vi "Dashboard Main.vi"() -> ()   [LabVIEW 2019]
uses:
  <vilib>/Utility/miscctls.llb/LVRowAndColumnTypeDef.ctl
  <vilib>/event_ctls.llb/eventvkey.ctl
  <vilib>/Rock Robotics/Network Tables/NT Read Numeric Array.vi
  <vilib>/Rock Robotics/Network Tables/NT Read Boolean.vi
  <vilib>/Rock Robotics/WPI/Dashboard/WPI_DashboardLogging Global.vi
panel:
  in  "Camera Settings Right":T1={"Frame Rate"=30, "Compression"=30, "Size"=1, "DB Camera Config"=FALSE} {"Frame Rate" scale=1.0..30.0; "Compression" scale=100.0..-1.0; "Size" items=["640x480", "320x240", "160x120"]}
  in  "Camera Name Right":string(combo)="No Camera Selection"
  out "Camera Perf":string
  in  "Camera Settings":T1={"Frame Rate"=30, "Compression"=30, "Size"=1, "DB Camera Config"=FALSE} {"Frame Rate" scale=1.0..30.0; "Compression" scale=100.0..-1.0; "Size" items=["640x480", "320x240", "160x120"]}
  in  "TCP":refnum<k5>
  in  "Rec Mode":enum32{"Stop", "Record", "Playback"}(radio)
  out "Robot IP":string
  out "Image Message":string="Timeout in Camera Communications"
  in  "Dashboard Tab":T2(tab)=enum."Custom"
  in  "Select Auto":string(combo)="Select Autonomous ..."
  out "NT Connection":bool
  out "MotorChart R":cluster{"Numeric":dbl, "Numeric":dbl}(graph)
  out "MotorChart L":cluster{"Numeric":dbl, "Numeric":dbl}(graph)
  out "MotorSliders R":cluster{"MotorSlide1":dbl, "MotorSlide2":dbl} {"MotorSlide2" scale=-1.0..1.0 scale format="%#_2e"; "MotorSlide1" scale=-1.0..1.0 scale format="%#_2e"}
  out "MotorSliders L":cluster{"MotorSlide1":dbl, "MotorSlide2":dbl} {"MotorSlide2" scale=-1.0..1.0 scale format="%#_2e"; "MotorSlide1" scale=-1.0..1.0 scale format="%#_2e"}
  out "Gyro":dbl(knob) scale=0.0..360.0
  out "JS1 Z":dbl(slide) scale=-1.0..1.0 scale format="%#_2e"
  out "JS1 Graph":cluster{"X":dbl, "Y":dbl}[](graph)
  out "JS1 Buttons":T3
  out "JS2 Z":dbl(slide) scale=-1.0..1.0 scale format="%#_2e"
  out "JS2 Graph":cluster{"X":dbl, "Y":dbl}[](graph)
  out "JS2 Buttons":T3
  out "Mode":T4(ring)=enum."Auto Disabled"
  out "Right Camera Perf":cluster{"Bandwidth (Mbps)":dbl, "FPS":dbl}
  out "Camera Image Right":T5(plugin-control)
  in  "DB/String 9":string
  in  "DB/String 8":string
  in  "DB/String 7":string
  in  "DB/String 6":string
  in  "DB/String 5":string
  in  "DB/String 4":string
  in  "DB/String 3":string
  in  "DB/String 2":string
  in  "DB/String 1":string
  in  "DB/String 0":string
  in  "DB/Slider 0":dbl(slide) scale=0.0..5.0
  in  "DB/Slider 1":dbl(slide) scale=0.0..5.0
  in  "DB/Slider 2":dbl(slide) scale=0.0..5.0
  in  "DB/Slider 3":dbl(slide) scale=0.0..5.0
  out "DB/LED 3":bool
  out "DB/LED 2":bool
  out "DB/LED 1":bool
  out "DB/LED 0":bool
  in  "DB/Button 3":bool
  in  "DB/Button 2":bool
  in  "DB/Button 1":bool
  in  "DB/Button 0":bool caption="New Name"
  in  "X-HAIR":bool
  out "Ball for shooter":bool caption="Ball ready"
  in  "RETICLE SHAPE":bool caption="RET SHAPE"
  in  "Color":u32(colorbox)=16775210
  out "Intake rotation":dbl(knob) scale=-100.0..100.0
  out "version_note":string
  in  "FIRE PULSE":dbl=0.4 caption="PULSE (s)" min=0.1 max=1.0 step=0.05 format="%#.1g"
  in  "FIRE SPD":dbl=0.4 min=0.4 max=1.0 step=0.1 format="%#.1g"
  out "GAME COLOR":u32(colorbox)
  out "SENSOR COLOR":u32(colorbox)
  out "DRIVER Z":dbl
  out "DRIVER Y":dbl
  out "SHOOTER HT":dbl[](array[slide]) caption="SHOOTER Ht & Spd" scale=0.2..1.0
  out "CW ROTATION":bool
  out "CW DEPLOY":bool
  out "LIFT LOCK":bool
  out "INV DRIVE":bool
  out "FORZA":bool
  out "1 Joystick":bool
  out "NEO MOTOR TEMPS":dbl[](array[slide])=[106.99300699300699] scale=50.0..200.0
  in  "HEIGHT":i32=20
  in  "TOP":i32=130
  in  "WIDE":i32=40
  in  "LEFT":i32=140
  in  "Test Slider":dbl(slide) scale=0.0..100.0 scale format="%#_3g"
  in  "On/Off":bool caption="Solenoid"
  in  "Test Name":u16(ring) items=["Select the test to run..."]
  in  "Test Tree":string(tree)
  in  "Motor":cluster{"Value":dbl, "Enable":bool} {"Value" scale=-1.0..1.0 scale format="%#_3g"}
  out "Progress":T6 {"Test Progress" scale=0.0..100.0}
  in  "Rev/Fwd":cluster{"Forward":bool, "Reverse":bool}
  in  "Test Ring":u16(ring) items=["Monochrome", "Color"]
  out "Cmd Status":string
  in  "Execute Command":bool
  in  "Command Params":string[][](table)
  in  "Command Selection":i32(listbox)
  in  "CheckList":i32(listbox)
  out "Tree":string(tree)
  out "Camera Image":T5(plugin-control)
  out "Background":bool
  in  "Camera Name":string(combo)="No Camera Selection"
  # "HW"
  # "HW"
  # "Joysticks"
  # "Drive Motors"
  # "Front"
  # "Right"
  # "Left"
  # "Back"
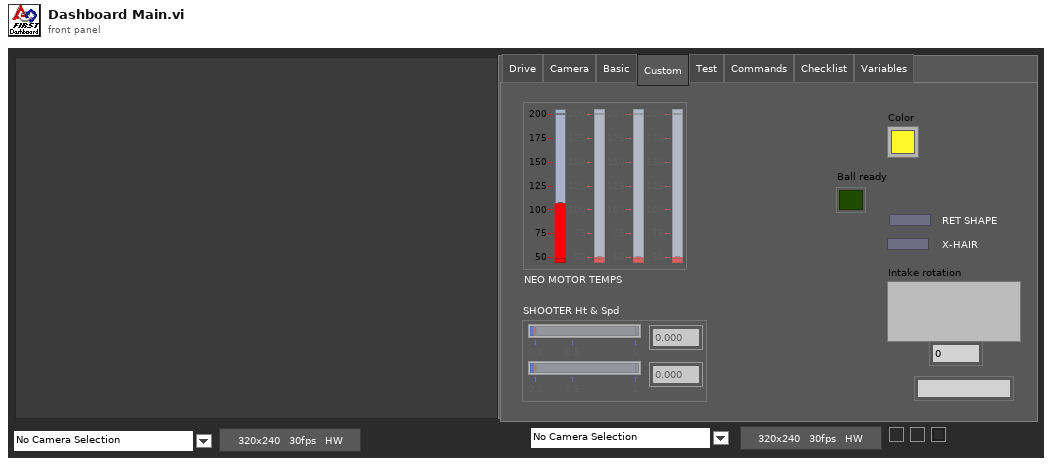
[diagram p1: front panel]
types:
  T1 = cluster{"Frame Rate":i32, "Compression":i32, "Size":u16, "DB Camera Config":bool}
  T2 = enum32{"Drive", "Camera", "Basic", "Custom", "Test", "Commands", "Checklist", "Variables"}
  T3 = cluster{bool, bool, bool, bool, bool, bool, bool, bool, bool, bool, bool, bool}
  T4 = enum8{"Tele-Op Disabled", "Tele-Op Enabled", "Auto Disabled", "Auto Enabled", "Test Disabled", "Test Enabled", "Disconnected", "No Code", "E-Stop"}
  T5 = typedef "IMAQ Image.ctl" = refnum<image>
  T6 = cluster{"Test Progress":u8, "Test Progress Text":string}
  T7 = cluster{"Save Path":path, "Interval (s)":dbl, "Keep":i32}
  T8 = typedef "Image Type" = u32
  T9 = cluster{"IDs":cluster{"RPC field ID":u16, "Unique ID":u16}, "String":string}
  T10 = cluster{"Error Strings":string, "Disable Counts":cluster{u16, u16}, "Rail Faults":cluster{u16, u16, u16}, "Robot IP":string, "DB Mode":u8, "Event Info":cluster{"Name":string, "Type":u8, "Number":u16, "Replay":u8}}
  T11 = cluster{"Storage":cluster{"Disk Free":u64, "RAM Block":u32, "RAM free":u32}, "CPU Utilization":cluster{"CPU % ISR":sgl, "CPU % Time Crit":sgl, "CPU % Timed Str":sgl, "CPU % High":sgl, "CPU % Above":sgl, "CPU % Normal":sgl, "CPU % Low":sgl}, "CAN":cluster{"% Bus Utilization":sgl, "Bus Off Cnt":u32, "TX_FIFO Full Cnt":u32, "Receive Error Cnt":u8, "Transmit Error Cnt":u8}, "HID":cluster{"HID Outputs":u32, "Rumble Low":u16, "Rumble High":u16}[]}
  T12 = cluster{"Status bits":cluster{"Test Mode":bool, "Autonomous":bool, "Enabled":bool, "Code Start":bool, "Brownout":bool, "Reserved 2":bool, "Reserved 3":bool, "E-Stop":bool}, "Code Trace":cluster{"Disabled":bool, "TeleOp":bool, "Auto":bool, "Test":bool}, "Controller Type":enum16{"unknown", "cRIO", "roboRio"}, "Code?":enum16{"unknown", "noCode", "code"}, "Battery V":dbl}
  T13 = cluster{"Control Bits":cluster{"TestMode":bool, "Autonomous":bool, "Enabled":bool, "FMS Present":bool, bool, bool, bool, "E-Stop":bool}, "Team Station ":u8, "Countdown":sgl, "Joystick Values":cluster{"Axes":dbl[], "Buttons":bool[], "POVs":i16[]}[]}
  T14 = cluster{"Axes":dbl[], "Buttons":bool[], "POVs":i16[]}[]
  T15 = cluster{"Axes":dbl[], "Buttons":bool[], "POVs":i16[]}
  T16 = cluster{"Buttons[0]":bool, "Buttons[1]":bool, "Buttons[2]":bool, "Buttons[3]":bool, "Buttons[4]":bool, "Buttons[5]":bool, "Buttons[6]":bool, "Buttons[7]":bool, "Buttons[8]":bool, "Buttons[9]":bool, "Buttons[10]":bool, "Buttons[11]":bool}
  T17 = cluster{"Camera Image":refnum<vi>, "Dashboard Tab":refnum<vi>, "Background":refnum<vi>, "Rec Mode":refnum<vi>, "Test Slider":refnum<vi>, "On/Off ":refnum<vi>, "Test Ring":refnum<vi>, "Rev/Fwd":refnum<vi>, "Test Name":refnum<vi>, "Motor":refnum<vi>, "Progress":refnum<vi>, "CheckList":refnum<vi>, "Tree":refnum<vi>, "Test Tree":refnum<vi>, "Command Params":refnum<vi>, "Command Selection":refnum<vi>, "Execute Command":refnum<vi>, "Cmd Status":refnum<vi>, "Camera Settings":refnum<vi>, "Camera Name":refnum<vi>, "Camera Perf":refnum<vi>, "Camera Settings Right":refnum<vi>, "Camera Name Right":refnum<vi>, "Camera Image Right":refnum<vi>}
  T18 = cluster{"Global Rectangle":i32[], "Contours":cluster{"Contour Type":u32, "ROI Type":u32, "Points":i32[]}[]}
  T19 = cluster{"Left":i32, "Top":i32, "Right":i32, "Bottom":i32}
  T20 = cluster{"Camera Name":string, string, "Saved DB Images Info":cluster{"Save Path":path, "Interval (s)":dbl, "Keep":i32}}
  T21 = cluster{"Camera Name Right":string, string, "Saved DB Images Info":cluster{"Save Path":path, "Interval (s)":dbl, "Keep":i32}}
  T22 = cluster{"Operation":enum16{"Update", "Clear"}, "Color Box":u32}[]
  T23 = typedef "eventvkey.ctl" = enum16{"ASCII", "Enter", "Return", "Shift", "Ctrl", "Alt", "Cmd", "Opt", "Caps", "NumLock", "Clear", "Break", "Up", "Down", "Left", "Right", "Insert", "Delete", "Home", "End", "PageUp", "PageDown", "Escape", "Help", "Pause", "ScrollLock", "F1", "F2", "F3", "F4", "F5", "F6", "F7", "F8", "F9", "F10", "F11", "F12", "F13", "F14", "F15", "F16", "F17", "F18", "F19", "F20", "F21", "F22", "F23", "F24", "Play", "VolumeUp", "VolumeDown", "Mute", "Two Byte Char"}
  T24 = cluster{"Image Size":bool, "Image Type":bool, "Pixel Value":bool, "ROI Information":bool, "Zoom Factor":bool}
  T25 = cluster{"Operation":enum16{"Update", "Clear"}, "Color Box":u32}
  T26 = typedef "LVRowAndColumnTypeDef.ctl" = cluster{"Row":i32, "Column":i32}
  T27 = cluster{"Shift":bool, "Ctrl":bool, "Alt":bool, "Cmd":bool, "Opt":bool}
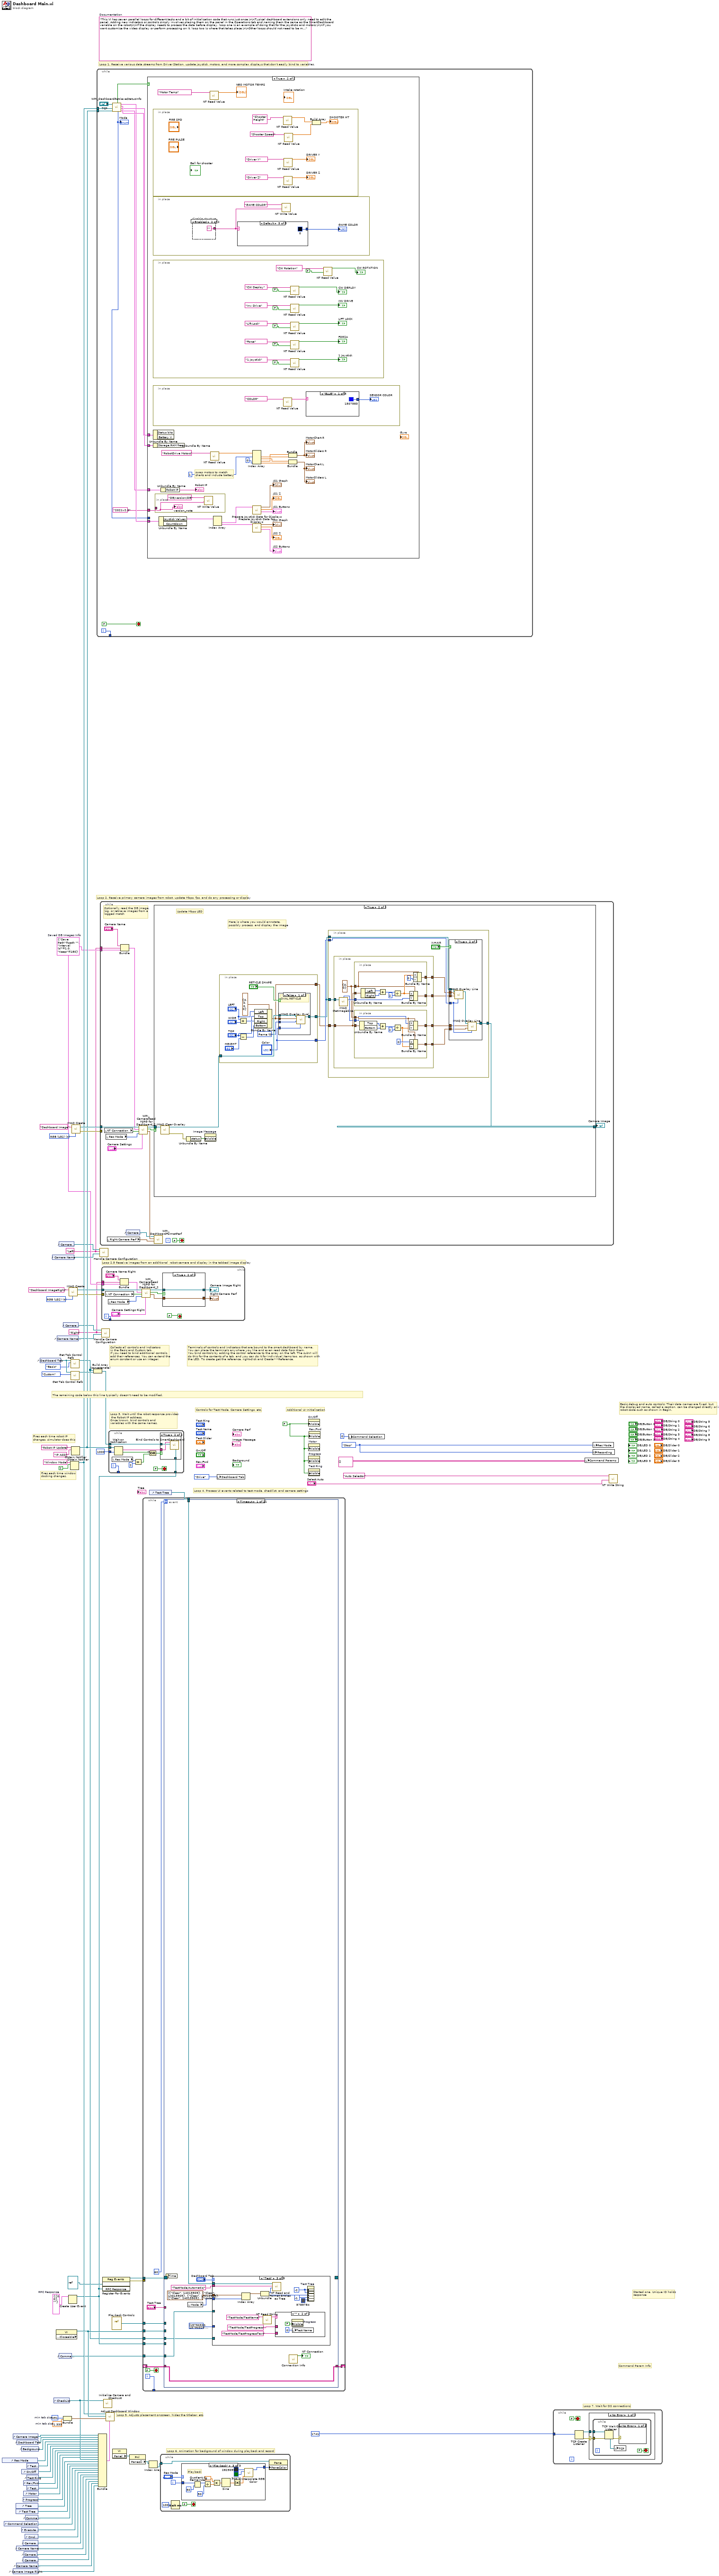
[diagram p0: block diagram]
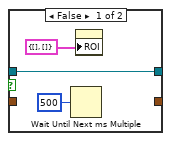
[diagram p2: hidden frame]
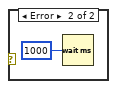
[diagram p3: hidden frame]
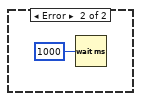
[diagram p4: hidden frame]
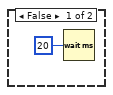
[diagram p5: hidden frame]
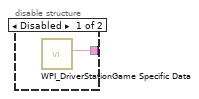
[diagram p6: hidden frame]
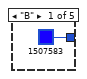
[diagram p7: hidden frame]
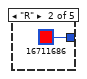
[diagram p8: hidden frame]
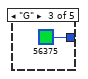
[diagram p9: hidden frame]
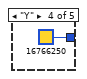
[diagram p10: hidden frame]
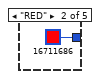
[diagram p11: hidden frame]
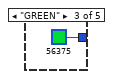
[diagram p12: hidden frame]
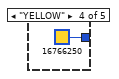
[diagram p13: hidden frame]
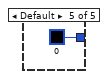
[diagram p14: hidden frame]
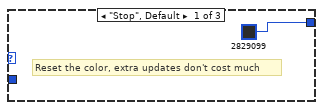
[diagram p15: hidden frame]
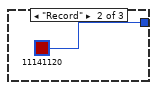
[diagram p16: hidden frame]
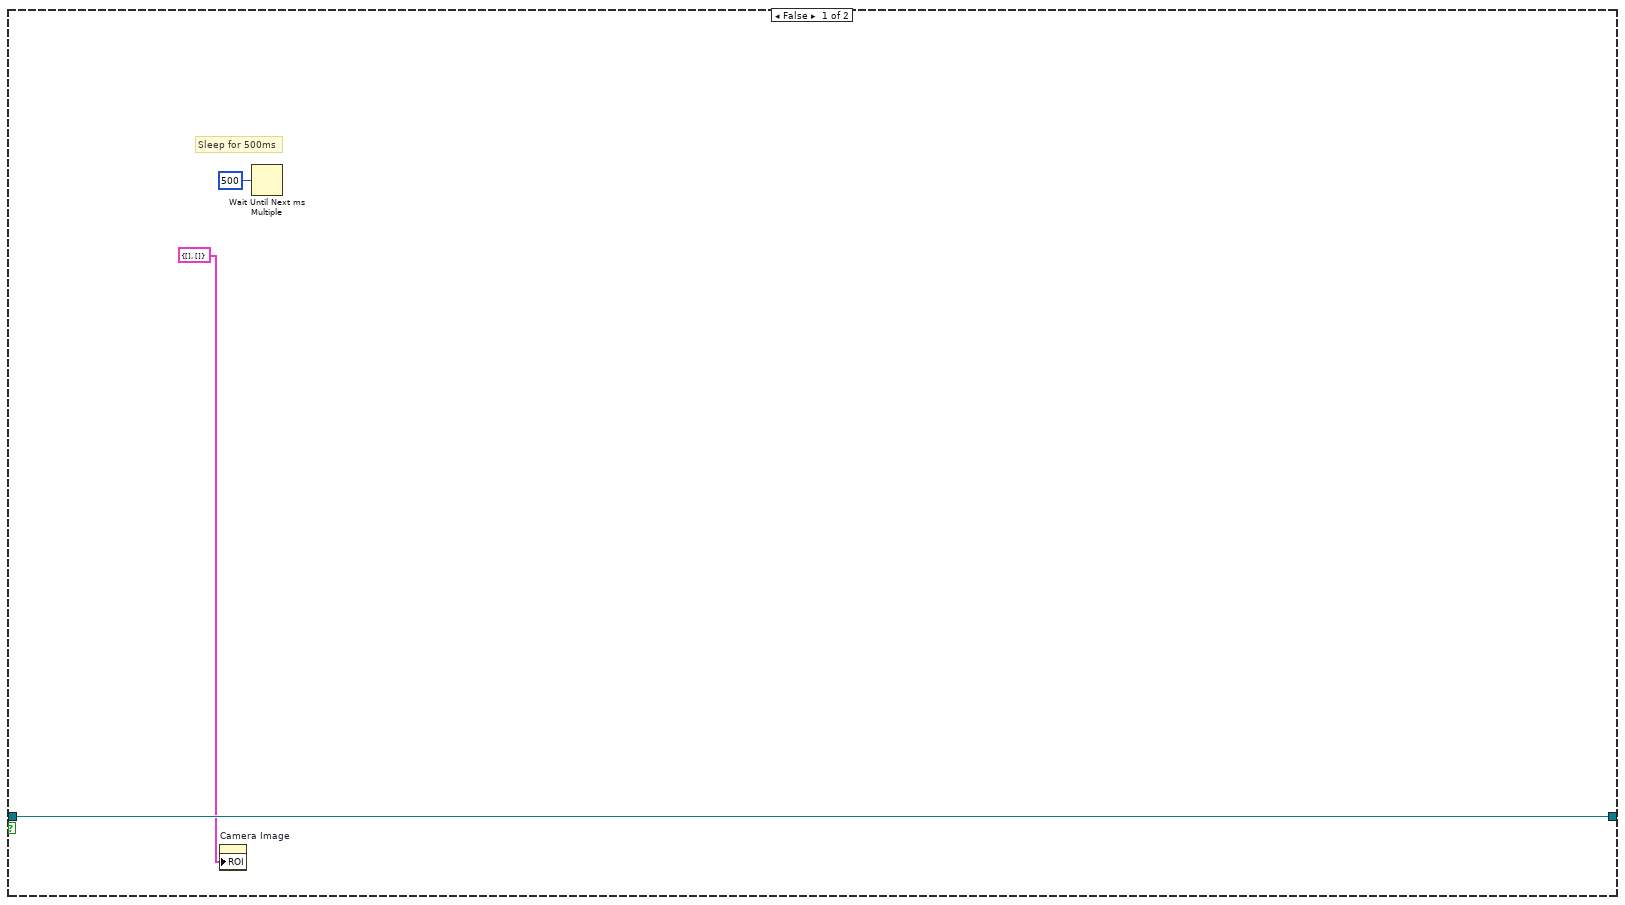
[diagram p18: hidden frame]
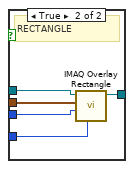
[diagram p20: hidden frame]
diagram:
  w3 = T7 {"Save Path"=path "", "Interval (s)"=1.0, "Keep"=180}  # Saved DB Images Info
  w2 = "Right"
  w1 = "Left"
  w13 = T8 4 items=["Grayscale (U8)", "Grayscale (I16)", "Grayscale (SGL)", "Complex (CSG)", "RGB (U32)", "HSL (U32)", "RGB (U64)"] ("Image Type")
  w29 = T9 {"IDs"={"RPC field ID"=0, "Unique ID"=0}, "String"=""}  # RPC Response
  w52 = 491  # min tab size
  w51 = 1.333  # min tab size
  w59 = enum32{"Stop", "Record", "Playback"}."Stop" ("Rec Mode")
  w36 = FALSE ("Visible")
  (unwired) "This VI has seven parallel loops for different tasks and a bit of initialization code that runs just once.\n\nTypical dashboard extensions only need to edit the panel. Adding new indicators or controls simply involves placing them on the panel in the Operations tab and naming them the same as the SmartDashboard variable on the robot\n\nIf the display needs to process the data before display, loop one is an example of doing that for the joysticks and motors.\n\nIf you want customize the video display or perform processing on it, loop two is where that takes place.\n\nOther loops should not need to be modified. They are pretty standard, and document the task they perform."  # Documentation
  w76 = T8 4 items=["Grayscale (U8)", "Grayscale (I16)", "Grayscale (SGL)", "Complex (CSG)", "RGB (U32)", "HSL (U32)", "RGB (U64)"] ("Image Type")
  # "Loop 2.5 Receive images from an additional  robot camera and display in the tabbed image display"
  # "Command Param Info"
  # "Started one, Unique ID holds\nresponse"
  # "Loop 7. Wait for DS connections"
  # "Basic debug and auto controls: Their data names are fixed, but\nthe displayed name, called a caption, can be changed directly or in\nrobot code such as shown in Begin."
  # "Controls for Test Mode, Camera Settings, etc."
  # "Additional UI Initialization"
  # "Loop 6. Animation for background of window during playback and record"
  # "Fires each time robot IP\nchanges, simulator does this"
  # "Fires each time window\ndocking changes."
  # "Collects all controls and indicators\nin the Basic and Custom tab.\nIf you need to bind additional controls,\nadd their references. You can extend the\nenum constant or use an integer."
  # "The remaining code below this line typically doesn't need to be modified."
  # "Loop 4. Process UI events related to test mode, checklist, and camera settings"
  # "Terminals of controls and indicators that are bound to the smart dashboard by name.\nYou can place the terminals anywhere you like and even read data from them.\nYou bind controls by adding the control reference to the array on the left. The subVI will\ndo this for the contents of a tab, and you can do it for individual items too, as shown with\nthe LED. To create get the reference, right-click and Create>>Reference."
  # "Loop 3. Wait until the robot response provides\n the Robot IP address.\nOnce known, bind controls and\nvariables with the same names."
  # "Loop 5. Adjusts placement onscreen, hides the titlebar, etc."
  # "Loop 1. Receive various data streams from Driver Station, update joystick, motors, and more complex displays that don't easily bind to variables."
  # "Loop 2. Receive primary camera images from robot, update Mbps, fps, and do any processing or display"
  n1 = control-ref of="Rec Mode"() -> (w42:refnum<vi>)
  n2 = control-ref of="Command Selection"() -> (w28:refnum<vi>)
  n3 = control-ref of="Camera Image Right"() -> (w6:refnum<vi>)
  n4 = control-ref of="Camera Image"() -> (w54:refnum<vi>)
  n5 = control-ref of="Tree"() -> (w46:refnum<vi>)
  n6 = control-ref of="Test Tree"() -> (w45:refnum<vi>)
  n7 = control-ref of="Camera Name"() -> (w19:refnum<vi>)
  n8 = control-ref of="Camera Name Right"() -> (w7:refnum<vi>)
  n9 = control-ref of="Dashboard Tab"() -> (w53:refnum<vi>)
  n10 = control-ref of="Execute Command"() -> (w30:refnum<vi>)
  n11 = control-ref of="Background"() -> (w49:refnum<vi>)
  n12 = control-ref of="On/Off"() -> (w40:refnum<vi>)
  n13 = control-ref of="Progress"() -> (w37:refnum<vi>)
  n14 = control-ref of="Camera Settings"() -> (w20:refnum<vi>)
  n15 = control-ref of="Camera Settings Right"() -> (w8:refnum<vi>)
  n16 = control-ref of="Rev/Fwd"() -> (w38:refnum<vi>)
  n17 = control-ref of="Motor"() -> (w43:refnum<vi>)
  n18 = control-ref of="Camera Perf"() -> (w18:refnum<vi>)
  n19 = control-ref of="Cmd Status"() -> (w24:refnum<vi>)
  n20 = control-ref of="Command Params"() -> (w31:refnum<vi>)
  n21 = control-ref of="Test Slider"() -> (w41:refnum<vi>)
  n22 = control-ref of="Test Ring"() -> (w39:refnum<vi>)
  n23 = control-ref of="Test Name"() -> (w44:refnum<vi>)
  n24 = control-ref of="Dashboard Tab"() -> (w57:refnum<vi>)
  n25 = control-ref of="Camera Name"() -> (w21:refnum<vi>)
  n26 = control-ref of="CheckList"() -> (w47:refnum<vi>)
  n27 = property class="VI" props=["Front Panel.Closeable"]() -> (reference out=w58:refnum<vi>)  [unwired: 2 in, 2 out]
  n28 = control-ref of="Camera Name Right"() -> (w9:refnum<vi>)
  n29 = control-ref of="Camera Settings"() -> (w22:refnum<vi>)
  n30 = control-ref of="Command Params"() -> (w23:refnum<vi>)
  n31 = control-ref of="Camera Settings Right"() -> (w10:refnum<vi>)
  n32 = Bundle("min tab size"=w52, "min tab size"=w51) -> (w50:cluster{"min tab size":i32, "min tab size":dbl})  [unwired: 1 in]
  n33 = Create User Event(user event datatype=w29) -> (user event=w25:refnum<user-event>)  [unwired: 1 in, 1 out]
  n34 = call "IMAQ Create"("Image Name"="Dashboard ImageRight", "Image Type"=w13) -> ("New Image"=w12:T5, "error out"=w11:errorcluster)  [unwired: 2 in, 1 out]
  n35 = Obtain Notifier(name (unnamed)="Window Mode", notification data type=TRUE) -> (notifier out=w34:refnum<notifier>)  [unwired: 2 in, 2 out]
  n36 = call <vilib>:"Get Tab Control Refs.vi"("Page Index"=T2."Basic" ("Dashboard Tab"), "TabControl in"=w57) -> ("ControlsOnPage"=w17:refnum<vi>[])  [unwired: 9 in]
  n37 = call <vilib>:"Get Tab Control Refs.vi"("Page Index"=T2."Custom" ("Dashboard Tab"), "TabControl in"=w57) -> ("ControlsOnPage"=w56:refnum<vi>[])  [unwired: 9 in]
  n38 = Obtain Notifier(name (unnamed)="Robot IP Update", notification data type="IP Addr" ("name (unnamed)")) -> (notifier out=w35:refnum<notifier>)  [unwired: 2 in, 2 out]
  n39 = call "IMAQ Create"("Image Name"="Dashboard Image", "Image Type"=w76) -> ("New Image"=w74:T5, "error out"=w73:errorcluster)  [unwired: 2 in, 1 out]
  n40 = Build Array (concatenate)(w17, w56) -> (w55:refnum<vi>[])
  n41 = while {
    tunnel: [w87] -> _
    tunnel: w35 -> [w81]
    tunnel: w34 -> [w78]
    i -> [w87]
    stop <- FALSE stop-if-true
    n42 = call <vilib>:"WPI_DashboardRetrieveStatusInfo.vi"("Binding Refnum"=w81, "Window Mode Notifier"=w78, "TCP Cnx"="TCP") -> ("Power and Errors"=w82:T10, "Robot Metrics"=w85:T11, "Status Info"=w86:T12, "Control Info"=w83:T13, "Robot Mode"=w80:T4, "Process?"=w84:bool)  [unwired: 3 in]
    "Mode" <- w80
    n43 = case shown="True" w84 {
      tunnel: w86 -> [_ w116]
      tunnel: w85 -> [_ w115]
      tunnel: w83 -> [_ w114]
      tunnel: w82 -> [_ w113]
      tunnel: w80 -> [_ _]
      tunnel: "2021v2.0" ("version_note") -> [_ w92]
      frame False {
        n44 = Wait (ms)(milliseconds to wait=u32 20) -> ()  [unwired: 1 out]
      }
      frame True {
        # "swap motors to match\ncharts and include battery"
        n45 = in-place {
          n46 = call-poly <vilib>:"NT Read Value.vi"("Name"="Shooter Height") -> ("Numeric"=w140:dbl)  [unwired: 9 in, 1 out]
          n47 = call-poly <vilib>:"NT Read Value.vi"("Name"="Driver Y") -> ("Numeric"=→"DRIVER Y":dbl)  [unwired: 9 in, 1 out]
          n48 = call-poly <vilib>:"NT Read Value.vi"("Name"="Driver Z") -> ("Numeric"=→"DRIVER Z":dbl)  [unwired: 9 in, 1 out]
          n49 = call-poly <vilib>:"NT Read Value.vi"("Name"="Shooter Speed") -> ("Numeric"=w138:dbl)  [unwired: 9 in, 1 out]
          n50 = Build Array(w140, w138) -> (→"SHOOTER HT":dbl[])
        }
        n51 = in-place {
          n52 = disable-structure shown="Enabled" {
            disable-tunnel: [w122 "" ("Game Specific Data")] -> w119
            frame Disabled {
              n53 = call <vilib>:"WPI_DriverStationGame Specific Data.vi"() -> ("Game Specific Data"=w122:string)  [unwired: 11 in]
            }
            frame Enabled {
            }
          }
          n54 = case shown="Default" w119 {
            tunnel: [u32 1507583 ("SENSOR COLOR") u32 16711686 ("SENSOR COLOR") u32 56375 ("SENSOR COLOR") u32 16766250 ("SENSOR COLOR") u32 0 ("SENSOR COLOR")] -> w121
            frame "B" {
            }
            frame "R" {
            }
            frame "G" {
            }
            frame "Y" {
            }
            frame Default {
            }
          }
          "GAME COLOR" <- w121
          n55 = call-poly <vilib>:"NT Write Value.vi"("String"=w119, "Name"="GAME COLOR") -> ()  [unwired: 9 in, 1 out]
        }
        n56 = in-place {
          n57 = call-poly <vilib>:"NT Read Value.vi"("Default Value"=FALSE, "Name"="CW Deploy") -> ("Boolean"=→"CW DEPLOY":bool)  [unwired: 8 in, 1 out]
          n58 = call-poly <vilib>:"NT Read Value.vi"("Default Value"=FALSE, "Name"="Inv Drive") -> ("Boolean"=→"INV DRIVE":bool)  [unwired: 8 in, 1 out]
          n59 = call-poly <vilib>:"NT Read Value.vi"("Default Value"=FALSE, "Name"="Lift Lock") -> ("Boolean"=→"LIFT LOCK":bool)  [unwired: 8 in, 1 out]
          n60 = call-poly <vilib>:"NT Read Value.vi"("Default Value"=FALSE, "Name"="Forza") -> ("Boolean"=→"FORZA":bool)  [unwired: 8 in, 1 out]
          n61 = call-poly <vilib>:"NT Read Value.vi"("Default Value"=FALSE, "Name"="1 Joystick") -> ("Boolean"=→"1 Joystick":bool)  [unwired: 8 in, 1 out]
          n62 = call-poly <vilib>:"NT Read Value.vi"("Default Value"=FALSE, "Name"="CW Rotation") -> ("Boolean"=→"CW ROTATION":bool)  [unwired: 8 in, 1 out]
        }
        n63 = in-place {
          n64 = call-poly <vilib>:"NT Read Value.vi"("Name"="COLOR") -> ("String"=w130:string)  [unwired: 9 in, 1 out]
          n65 = case shown="\"BLUE\"" w130 {
            tunnel: [u32 1507583 ("SENSOR COLOR") u32 16711686 ("SENSOR COLOR") u32 56375 ("SENSOR COLOR") u32 16766250 ("SENSOR COLOR") u32 0 ("SENSOR COLOR")] -> w129
            frame "BLUE" {
            }
            frame "RED" {
            }
            frame "GREEN" {
            }
            frame "YELLOW" {
            }
            frame Default {
            }
          }
          "SENSOR COLOR" <- w129
        }
        n66 = Unbundle By Name(w116) -> ()  [unwired: 2 out]
        n67 = Unbundle By Name(w115) -> ()  [unwired: 1 out]
        n68 = in-place {
          in-place-border: w92 -> [w117]
          n69 = call-poly <vilib>:"NT Write Value.vi"("String"=w117, "Name"="DB/version/DB") -> ()  [unwired: 9 in, 1 out]
          "version_note" <- w117
        }
        n70 = Unbundle By Name(w114) -> ("Joystick Values"=w104:T14)  [unwired: 1 out]
        n71 = Unbundle By Name(w113) -> ("Robot IP"=→"Robot IP":string)
        n72 = call-poly <vilib>:"NT Read Value.vi"("Name"="Motor Temp") -> ("Numeric Array"=→"NEO MOTOR TEMPS":dbl[])  [unwired: 9 in, 1 out]
        n73 = call-poly <vilib>:"NT Read Value.vi"("Name"="RobotDrive Motors") -> ("Numeric Array"=w94:dbl[])  [unwired: 9 in, 1 out]
        n74 = Index Array(array=w104) -> (element #1=w103:T15, element #2=w99:T15)  [unwired: 2 in]
        n75 = Index Array(array=w94, index #1=1, index #4=0) -> (element #1=w108:dbl, element #2=w109:dbl, element #3=w107:dbl, element #4=w112:dbl)  [unwired: 2 in]
        n76 = call "Prepare Joystick Data for Displays.vi"("Joystick Values"=w103) -> ("Buttons"=→"JS1 Buttons":T16, "Z Axis"=→"JS1 Z":dbl, "Cartesian Data"=→"JS1 Graph":cluster{"X axis":dbl, "X axis":dbl}[])  [unwired: 8 in]
        n77 = call "Prepare Joystick Data for Displays.vi"("Joystick Values"=w99) -> ("Buttons"=→"JS2 Buttons":T16, "Z Axis"=→"JS2 Z":dbl, "Cartesian Data"=→"JS2 Graph":cluster{"X axis":dbl, "X axis":dbl}[])  [unwired: 8 in]
        n78 = Bundle("Numeric"=w107, "Numeric"=w108) -> (→"MotorChart R" →"MotorSliders R":cluster{"Numeric":dbl, "Numeric":dbl})  [unwired: 1 in]
        n79 = Bundle("Numeric"=w109, "Numeric"=w112) -> (→"MotorChart L" →"MotorSliders L":cluster{"Numeric":dbl, "Numeric":dbl})  [unwired: 1 in]
      }
    }
  }
  n80 = Bundle("Camera Image"=w54, "Dashboard Tab"=w53, "Background"=w49, "Rec Mode"=w42, "Test Slider"=w41, "On/Off"=w40, "Test Ring"=w39, "Rev/Fwd"=w38, "Test Name"=w44, "Motor"=w43, "Progress"=w37, "CheckList"=w47, "Tree"=w46, "Test Tree"=w45, "Command Params"=w31, "Command Selection"=w28, "Execute Command"=w30, "Cmd Status"=w24, "Camera Settings"=w20, "Camera Name"=w19, "Camera Perf"=w18, "Camera Settings Right"=w8, "Camera Name Right"=w7, "Camera Image Right"=w6) -> (w48:T17)  [unwired: 1 in]
  n81 = call "Handle Camera Configuration.vi"("CameraNameRef"=w21, "Display Name"=w1, "ClusterRef"=w22) -> ()  [unwired: 9 in]
  n82 = while {
    tunnel: w74 -> [w177]
    tunnel: w73 -> [_]
    tunnel: w3 -> [w170]
    tunnel: w1 -> [w167]
    stop <- FALSE stop-if-true
    # "Optionally read the DB image,\nlog, or retrieve images from a\nlogged match"
    n83 = local read "NT Connection"() -> (w171:bool)
    n84 = local read "Rec Mode"() -> (w174:enum32{"Stop", "Record", "Playback"})
    n85 = local read "Right Camera Perf"() -> (w165:cluster{"Bandwidth (Mbps)":dbl, "FPS":dbl})
    n86 = Bundle("Camera Name"="Camera Name", w167, "Saved DB Images Info"=w170) -> (w169:T20)  [unwired: 1 in]
    n87 = control-ref of="Camera Perf"() -> (w164:refnum<vi>)
    n88 = call <vilib>:"WPI_CameraRead MJPG for Dashboard_2.vi"("Camera Settings"="Camera Settings", "Rec Mode"=w174, "NT Connection"=w171, "Capture Info"=w169, "Image in"=w177) -> ("perf info"=w166:cluster{"Bandwidth (Mbps)":dbl, "fps":dbl}, "Active"=w175:bool, "Image\\ out"=w176:T5)  [unwired: 4 in]
    n89 = case shown="True" w175 {
      tunnel: w176 -> [w180 w187]
      tunnel: [w180 w185] -> w172
      frame False {
        # "Sleep for 500ms"
        n90 = property on="Camera Image" class="ImageControl"("ROI"=T18 {"Global Rectangle"=[], "Contours"=[]}) -> ()  [unwired: 2 in, 2 out]
        n91 = Wait Until Next ms Multiple(millisecond multiple=u32 500) -> ()  [unwired: 1 out]
      }
      frame True {
        # "Here is where you would annotate,\npossibly process, and display the image"
        # "Update Mbps LED"
        n92 = call "IMAQ Clear Overlay"("Image"=w187) -> ("error out"=w188:errorcluster, "Image Out"=w186:T5)  [unwired: 2 in, 7 out]
        n93 = Unbundle By Name(w188) -> ("status"=w189:bool)
        n94 = property on="Image Message" class="Str"("Visible"=w189) -> ()  [unwired: 2 in, 2 out]
        n95 = in-place {
          in-place-border: w186 -> [w252]
          in-place-border: [w251] -> w183
          in-place-border: ["Color"] -> w184
          in-place-border: [w240] -> w182
          w250 = u32 0 items=["Frame", "Fill"] ("Drawing Mode (Frame)")
          n96 = Add(x="LEFT", y="WIDE") -> (x+y=w249:i32)
          n97 = Subtract(x="TOP", y="HEIGHT") -> (x-y=w248:i32)
          n98 = Bundle By Name(cluster=T19 {"Left"=0, "Top"=0, "Right"=0, "Bottom"=0} ("Bounding Rectangle"), "Left"="LEFT", "Top"="TOP", "Right"=w249, "Bottom"=w248) -> (w240:T19)
          n99 = case shown="False" "RETICLE SHAPE" {
            tunnel: w252 -> [w256 w262]
            tunnel: [w257 w261] -> w251
            tunnel: w250 -> [w254 w260]
            tunnel: w240 -> [w255 w259]
            tunnel: "Color" -> [w253 w258]
            frame False {
              # "OVAL RETICLE"
              n100 = call "IMAQ Overlay Oval"("Color"=w253, "Drawing Mode (Frame)"=w254, "Bounding Rectangle"=w255, "Image"=w256) -> ("Image Out"=w257:T5)  [unwired: 6 in, 1 out]
            }
            frame True {
              # "RECTANGLE"
              n101 = call "IMAQ Overlay Rectangle"("Color"=w258, "Drawing Mode (Frame)"=w260, "Rectangle"=w259, "Image"=w262) -> ("Image Out"=w261:T5)  [unwired: 6 in, 1 out]
            }
          }
        }
        n102 = in-place {
          in-place-border: w183 -> [w198]
          in-place-border: [w197] -> w185
          in-place-border: w184 -> [w196]
          in-place-border: w183 -> [w195]
          in-place-border: w182 -> [w194]
          n103 = in-place {
            in-place-border: w195 -> [w208]
            in-place-border: w194 -> [w203]
            in-place-border: [w207] -> w193
            in-place-border: [w205] -> w192
            in-place-border: [w201] -> w191
            in-place-border: [w200] -> w190
            w204 = cluster{"X":i32, "Y":i32} {"X"=0, "Y"=0} ("Start Point")
            n104 = call "IMAQ GetImageSize"("Image"=w208) -> ("Y Resolution"=w206:i32, "X Resolution"=w202:i32)  [unwired: 3 in, 1 out]
            n105 = in-place {
              in-place-border: w203 -> [w230]
              in-place-border: [w224] -> w207
              in-place-border: w204 -> [w220]
              in-place-border: w206 -> [w222]
              in-place-border: [w221] -> w205
              n106 = Unbundle By Name(w230) -> ("Left"=w229:i32, "Right"=w228:i32)
              n107 = Add(x=w229, y=w228) -> (x+y=w227:i32)
              n108 = Divide(x=w227, y=2) -> (x/y=w223:dbl)
              n109 = Bundle By Name(cluster=w220, "X"=w223, "Y"=w222) -> (w221:cluster{"X":i32, "Y":i32})
              n110 = Bundle By Name(cluster=w220, "X"=w223, "Y"=0) -> (w224:cluster{"X":i32, "Y":i32})
            }
            n111 = in-place {
              in-place-border: w203 -> [w219]
              in-place-border: [w214] -> w200
              in-place-border: w204 -> [w212]
              in-place-border: [w213] -> w201
              in-place-border: w202 -> [w209]
              n112 = Unbundle By Name(w219) -> ("Top"=w218:i32, "Bottom"=w217:i32)
              n113 = Add(x=w218, y=w217) -> (x+y=w216:i32)
              n114 = Divide(x=w216, y=2) -> (x/y=w210:dbl)
              n115 = Bundle By Name(cluster=w212, "X"=w209, "Y"=w210) -> (w213:cluster{"X":i32, "Y":i32})
              n116 = Bundle By Name(cluster=w212, "X"=0 ("Y"), "Y"=w210) -> (w214:cluster{"X":i32, "Y":i32})
            }
          }
          n117 = case shown="True" "X-HAIR" {
            tunnel: w198 -> [w231 w238]
            tunnel: [w231 w235] -> w197
            tunnel: w196 -> [_ w234]
            tunnel: w193 -> [_ w237]
            tunnel: w192 -> [_ w236]
            tunnel: w191 -> [_ w233]
            tunnel: w190 -> [_ w232]
            frame False {
            }
            frame True {
              n118 = call "IMAQ Overlay Line"("Color"=w234, "End Point"=w236, "Start Point"=w237, "Image"=w238) -> ("Image Out"=w239:T5)  [unwired: 6 in, 1 out]
              n119 = call "IMAQ Overlay Line"("Color"=w234, "End Point"=w232, "Start Point"=w233, "Image"=w239) -> ("Image Out"=w235:T5)  [unwired: 6 in, 1 out]
            }
          }
        }
      }
    }
    "Camera Image" <- w172
    n120 = call <vilib>:"WPI_DashboardFormatPerf.vi"("Right Camera Perf"=w165, "Performance"=w166, "String in"=w164) -> ()  [unwired: 9 in]
  }
  n121 = call "Handle Camera Configuration.vi"("CameraNameRef"=w9, "Display Name"=w2, "ClusterRef"=w10) -> ()  [unwired: 9 in]
  n122 = while {
    tunnel: w12 -> [w277]
    tunnel: w11 -> [_]
    tunnel: [w272] -> _
    tunnel: w3 -> [w268]
    tunnel: w2 -> [w265]
    i -> [w272]
    stop <- FALSE stop-if-true
    n123 = local read "NT Connection"() -> (w269:bool)
    n124 = local read "Rec Mode"() -> (w276:enum32{"Stop", "Record", "Playback"})
    n125 = Bundle("Camera Name Right"="Camera Name Right", w265, "Saved DB Images Info"=w268) -> (w267:T21)  [unwired: 1 in]
    n126 = call <vilib>:"WPI_CameraRead MJPG for Dashboard_2.vi"("Camera Settings"="Camera Settings Right", "Rec Mode"=w276, "NT Connection"=w269, "Capture Info"=w267, "Image in"=w277) -> ("perf info"=w263:cluster{"Bandwidth (Mbps)":dbl, "fps":dbl}, "Active"=w271:bool, "Image\\ out"=w274:T5)  [unwired: 4 in]
    n127 = case shown="True" w271 {
      tunnel: w274 -> [w279 w282]
      tunnel: [w279 w282] -> w270
      tunnel: [_ w281] -> w264
      tunnel: w263 -> [_ w281]
      frame False {
        n128 = Wait Until Next ms Multiple(millisecond multiple=u32 500) -> ()  [unwired: 1 out]
        n129 = property on="Camera Image Right" class="ImageControl"("ROI"=T18 {"Global Rectangle"=[], "Contours"=[]}) -> ()  [unwired: 2 in, 2 out]
      }
      frame True {
      }
    }
    "Camera Image Right" <- w270
    "Right Camera Perf" <- w264
  }
  n130 = register-events(refnum<vi> refnum, w25) -> (reference out=w63:refnum<event-registration>, error out=w62:errorcluster)  [unwired: 2 in]
  n131 = call "Initialize Camera and CheckList.vi"("ListBox in"=w47) -> ()  [unwired: 11 in]
  n132 = call "Adjust Dashboard Window.vi"("Sizing Refnums"=w48, "Size Constraints"=w50, "VI"=w58, "WIn Mode"=w34) -> ()  [unwired: 8 in]
  n133 = while {
    tunnel: w55 -> [w294]
    tunnel: w35 -> [w292]
    tunnel: [w290] -> _
    tunnel: u32 1000 ("milliseconds to wait") -> [w289]
    tunnel: w25 -> [w283]
    i -> [w290]
    stop <- FALSE stop-if-true
    n134 = local read "Rec Mode"() -> (w285:enum32{"Stop", "Record", "Playback"})
    n135 = Wait on Notification(notifier=w292, timeout in ms (-1)=w289) -> (notification=w291:string, timed out?=w287:bool)  [unwired: 2 in, 2 out]
    n136 = Equal?(x=w285, y=u16 2 ("Rec Mode")) -> (x = y?=w286:bool)
    n137 = Compound Arithmetic op=OR(invert w287, w286) -> (w288:bool)
    n138 = case shown="True" w288 {
      tunnel: w294 -> [_ w297]
      tunnel: w291 -> [_ w296]
      tunnel: w283 -> [_ w295]
      frame False {
      }
      frame True {
        n139 = call <vilib>:"Bind Controls to SmartDashboard.vi"("RPC ref"=w295, "Bound Control Refs"=w297, "Server IP Address"=w296) -> ()  [unwired: 9 in]
      }
    }
  }
  n140 = vi-ref "Playback Controls.vi"() -> (w64:refnum<vi>)
  n141 = property class="VI"() -> ("Panel"=w66:refnum<vi>)  [unwired: 2 in, 2 out]
  n142 = property class="Pnl"(reference=w66) -> ("Panes[]"=w67:refnum<vi>[])  [unwired: 1 in, 2 out]
  n143 = Index Array(array=w67) -> (element=w65:refnum<vi>)  [unwired: 1 in]
  n144 = control-ref of="Test Tree"() -> (w68:refnum<vi>)
  n145 = while {
    tunnel: [w307] -> _
    tunnel: w68 -> [w306]
    tunnel: w64 -> [w305]
    tunnel: w63 -> [w304]
    tunnel: w62 -> [_]
    tunnel: w58 -> [w303]
    tunnel: w25 -> [w302]
    tunnel: w23 -> [w301]
    shift-right: [w300] -> _
    shift-left: _ -> [w299]
    tunnel: w17 -> [w298]
    i -> [w307]
    stop <- FALSE stop-if-true
    n146 = event shown="[0] Timeout" {
      selector: w304 -> [_ _ _ _ _ _ _ _ _ _ _ _ _ _ _ _ _ _ _ _ _]
      dyn-events: [_ _ _ _ _ _ _ _ _ _ _ _ _ _ _ _ w567 _ _ _ _] -> _
      timeout: u32 60 ("milliseconds to wait") -> [_ _ _ _ _ _ _ _ _ _ _ _ _ _ _ _ _ _ _ _ _]
      tunnel: w306 -> [w319 _ _ _ _ _ _ _ _ _ _ _ _ _ _ _ _ _ _ _ _]
      tunnel: "Test Tree" -> [_ _ _ _ _ _ _ _ _ _ _ w534 w542 w544 w548 w556 _ _ _ _ _]
      tunnel: w305 -> [_ _ _ _ _ _ _ _ _ _ _ _ _ _ _ _ w569 _ w587 _ _]
      tunnel: w303 -> [_ _ _ _ _ _ _ _ _ _ _ _ _ _ _ _ w565 _ _ _ _]
      tunnel: w302 -> [_ _ _ _ _ _ _ _ _ _ _ _ _ _ _ _ w563 _ _ _ _]
      tunnel: w301 -> [w314 _ _ _ _ _ w485 _ _ _ _ _ _ _ _ _ _ _ _ _ _]
      tunnel: [w313 w362 w464 w469 w478 w482 w483 w492 w502 w509 w521 w533 w540 w543 w547 w555 w562 w582 w584 w588 w601] -> w300
      tunnel: w299 -> [w313 w362 w464 w469 w478 w482 w483 _ _ w509 w521 w533 w540 w543 w547 w555 w562 w582 w584 w588 w601]
      tunnel: w298 -> [w311 _ _ _ _ _ _ _ _ _ _ _ _ _ _ _ _ _ _ _ _]
      event Timeout {
        n147 = event-data() -> ()  [unwired: 1 in, 1 out]
        n148 = local read "Mode"() -> (w316:T4)
        n149 = case shown="\"Test\"" "Dashboard Tab" {
          tunnel: w319 -> [_ _ w335 _ _]
          tunnel: "TestMode/Automatic/" ("Name Pattern") -> [_ _ w334 _ _]
          tunnel: T22 [{"Operation"=enum."Clear", "Color Box"=14013909}, {"Operation"=enum."Clear", "Color Box"=14013909}, {"Operation"=enum."Clear", "Color Box"=14013909}, {"Operation"=enum."Clear", "Color Box"=14013909}, {"Operation"=enum."Update", "Color Box"=14013909}, {"Operation"=enum."Update", "Color Box"=16777215}, {"Operation"=enum."Clear", "Color Box"=14013909}, {"Operation"=enum."Clear", "Color Box"=14013909}, {"Operation"=enum."Clear", "Color Box"=14013909}] -> [_ _ w327 _ w355]
          tunnel: w316 -> [_ _ w326 _ w354]
          tunnel: u32[] [15790320, 15790320, 15790320, 15790320, 16777215, 16777215, 15790320, 15790320, 15790320] -> [_ _ _ _ w360]
          tunnel: w314 -> [_ _ _ _ w348]
          tunnel: w311 -> [_ w321 _ _ _]
          frame "Custom", Default {
          }
          frame "Basic" {
            n150 = call <vilib>:"WPI_DashboardUpdateNames.vi"("Controls on Tab"=w321) -> ()  [unwired: 11 in]
          }
          frame "Test" {
            w333 = -2 ("Active Item:Row Number")
            n151 = Index Array(array=w327, index=w326) -> (element=w328:T25)
            n152 = Unbundle(w328) -> ("Operation"=w329:enum16{"Update", "Clear"}, "Color Box"=w330:u32)
            n153 = call <vilib>:"NT Read String.vi"("Name"="TestMode/TestName") -> ("String"=w324:string)  [unwired: 9 in, 1 out]
            n154 = call <vilib>:"NT Read and Format Entries as Tree.vi"("Operation"=w329, "Name Pattern"=w334, "Tree Refnum"=w335) -> ()  [unwired: 7 in, 2 out]
            n155 = case shown="\"\"" w324 {
              tunnel: "TestMode/TestProgress" ("Name") -> [w337 _]
              tunnel: "TestMode/TestProgressText" ("Name") -> [w336 _]
              frame Default {
                n156 = call <vilib>:"NT Read Number.vi"("Name"=w337) -> ("Numeric"=w338:dbl)  [unwired: 9 in, 1 out]
                n157 = call <vilib>:"NT Read String.vi"("Name"=w336) -> ("String"=w339:string)  [unwired: 9 in, 1 out]
                n158 = Bundle("Numeric"=w338, "String"=w339) -> (→"Progress":cluster{"Numeric":dbl, "String":string})  [unwired: 1 in]
              }
              frame "" {
                n159 = property on="Progress" class="Clust (strict)"("Visible"=FALSE) -> ()  [unwired: 2 in, 2 out]
                n160 = local write "Test Name"(u16 0) -> ()
              }
            }
            n161 = property on="Test Tree" class="Tree (strict)"("Active Item Row Number"=w333, "ActiveColNum"=w333, "CellBG"=w330, "Active Item Row Number"=-1 ("Active Item:Row Number"), "CellBG"=u32 5789784 ("Color Box")) -> ()  [unwired: 2 in, 2 out]
          }
          frame "Variables" {
            w345 = string[] ["CameraPublisher", "Usage", "DB"]  # Items to initially close
            n162 = First Call?() -> (First Call?: T/F=w346:bool)
            n163 = control-ref of="Tree"() -> (w347:refnum<vi>)
            n164 = Select(t=w345, s=w346, f=string[] []) -> (s? t:f=w343:string[])
            n165 = call <vilib>:"NT Read and Format Entries as Tree.vi"("Tags to  Close"=w343, "Tree Refnum"=w347) -> ()  [unwired: 8 in, 2 out]
          }
          frame "Commands" {
            w356 = u32 5789784 ("Color Box")
            w357 = T26 {"Row"=-1, "Column"=-2} ("Active Cell:Active Cell")
            w359 = T26 {"Row"=-2, "Column"=-2} ("Active Cell:Active Cell")
            n166 = Index Array(array=w360, index=w354) -> (element=w358:u32)
            n167 = Index Array(array=w355, index=w354) -> (element=w353:T25)
            n168 = Unbundle(w353) -> ("Operation"=w352:enum16{"Update", "Clear"})  [unwired: 1 out]
            n169 = local read "Command Selection"() -> (w351:i32)
            n170 = property on="Command Selection" class="MCListbox (strict)"("ActiveCell"=w359, "CellBG"=w358, "ActiveCell"=w357, "CellBG"=w356) -> ()  [unwired: 2 in, 2 out]
            n171 = call <vilib>:"WPI_DashboardUpdate RPC Info.vi"("Operation"=w352) -> ("update"=w350:bool, "commands"=w349:string[][])  [unwired: 9 in]
            n172 = property on="Command Selection" class="MCListbox (strict)"("ItemNames"=w349) -> ()  [unwired: 2 in, 2 out]
            n173 = property on="Command Params" class="Tbl (strict)"("Active Cell"=w359, "Cell BG Color"=w358, "Active Cell"=w357, "Cell BG Color"=w356) -> ()  [unwired: 2 in, 2 out]
            n174 = call <vilib>:"WPI_DashboardUpdate Command Params.vi"("Update"=w350, "NewVal"=w351, "Commands"=w349, "Param Tbl"=w348) -> ()  [unwired: 7 in, 1 out]
          }
        }
        n175 = call <vilib>:"Connextion Info.vi"() -> ("Connected"=→"NT Connection":bool)  [unwired: 10 in, 1 out]
      }
      event "Test Tree": Value Change {
        # "Show appropriate\ncontrols"
        n176 = event-data() -> ("CtlRef"=w365:refnum<vi>, "NewVal"=w363:string)  [unwired: 1 in]
        n177 = call <vilib>:"WPI_UtilitiesGetTreeIOName.vi"("NewVal"=w363, "TreeControl in"=w365) -> ("I/O Name"=w366:string)  [unwired: 9 in]
        n178 = case shown="\"Camera\"" w366 {
          selector: w366 -> [_ w373 _ w395 w404 _]
          tunnel: w363 -> [_ _ w392 w394 _ w411]
          tunnel: cluster{string[]}[] [{["640x480", "320x240", "160x120"]}, {["Auto", "Fixed indoor", "Fixed outdoor 1", "Fixed outdoor 2", "Fixed fluorescent 1", "Fixed fluorescent 2", "Hold current"]}, {["Auto", "Flicker-free 50 Hz", "Flicker-free 60 Hz", "Hold current"]}, {["None", "Prioritize frame rate", "Prioritize image quality"]}, {["Monochrome", "Color"]}] -> [_ _ _ _ _ w410]
          frame Default {
            w368 = FALSE ("Visible")
            w367 = FALSE ("Visible")
            n179 = property on="Motor" class="Clust (strict)"("Visible"=w367) -> ()  [unwired: 2 in, 2 out]
            n180 = property on="Test Ring" class="Ring (strict)"("Visible"=w367) -> ()  [unwired: 2 in, 2 out]
            n181 = property on="Rev/Fwd" class="Clust (strict)"("Visible"=w368) -> ()  [unwired: 2 in, 2 out]
            n182 = property on="On/Off" class="Bool (strict)"("Visible"=w368) -> ()  [unwired: 2 in, 2 out]
            n183 = property on="Test Slider" class="Slide (strict)"("Visible"=w368) -> ()  [unwired: 2 in, 2 out]
          }
          frame "Analog Out", "Motor", "PWM" {
            w374 = FALSE ("Visible")
            n184 = case shown="\"Analog Out\"" w373 {
              tunnel: [1.0 ("Value") -1.0 ("Value") 0.0 ("Value")] -> w372
              tunnel: [255.0 ("Value") 1.0 ("Value") 5.0 ("Value")] -> w371
              tunnel: [128.0 ("Value") 0.0 ("Value") 0.0 ("Value")] -> w370
              tunnel: [64.0 ("Value") 0.5 ("Value") 1.0 ("Value")] -> w369
              frame "PWM" {
              }
              frame "Motor", Default {
              }
              frame "Analog Out" {
              }
            }
            n185 = property on="Motor" class="Clust (strict)"("Visible"=TRUE) -> ()  [unwired: 2 in, 2 out]
            n186 = property on="Value" class="Slide (strict)"("Value"=w370, "Scale.Minimum"=w372, "Scale.Maximum"=w371, "Scale.Increment"=w369) -> ()  [unwired: 2 in, 2 out]
            n187 = property on="On/Off" class="Bool (strict)"("Visible"=w374) -> ()  [unwired: 2 in, 2 out]
            n188 = property on="Test Slider" class="Slide (strict)"("Visible"=w374) -> ()  [unwired: 2 in, 2 out]
            n189 = property on="Test Ring" class="Ring (strict)"("Visible"=w374) -> ()  [unwired: 2 in, 2 out]
            n190 = property on="Rev/Fwd" class="Clust (strict)"("Visible"=w374) -> ()  [unwired: 2 in, 2 out]
          }
          frame "Servo" {
            w390 = FALSE ("Visible")
            n191 = call <vilib>:"NT Read Number.vi"("Name"=w392) -> ("Numeric"=w391:dbl)  [unwired: 9 in, 1 out]
            n192 = property on="Test Slider" class="Slide (strict)"("Visible"=TRUE, "Scale.Maximum"=170.0 ("Scale.Range:Maximum")) -> ()  [unwired: 2 in, 2 out]
            n193 = local write "Test Slider"(w391) -> ()
            n194 = property on="Motor" class="Clust (strict)"("Visible"=w390) -> ()  [unwired: 2 in, 2 out]
            n195 = property on="Rev/Fwd" class="Clust (strict)"("Visible"=w390) -> ()  [unwired: 2 in, 2 out]
            n196 = property on="On/Off" class="Bool (strict)"("Visible"=w390) -> ()  [unwired: 2 in, 2 out]
            n197 = property on="Test Ring" class="Ring (strict)"("Visible"=w390) -> ()  [unwired: 2 in, 2 out]
          }
          frame "Relay", "Solenoid" {
            w393 = FALSE ("Visible")
            n198 = property on="Motor" class="Clust (strict)"("Visible"=w393) -> ()  [unwired: 2 in, 2 out]
            n199 = property on="Test Slider" class="Slide (strict)"("Visible"=w393) -> ()  [unwired: 2 in, 2 out]
            n200 = Search and Replace String(input string=w394, search string="/Value  **", replace string="/Direction") -> (result string=w400:string)  [unwired: 5 in, 3 out]
            n201 = property on="Test Ring" class="Ring (strict)"("Visible"=w393) -> ()  [unwired: 2 in, 2 out]
            n202 = call <vilib>:"NT Read String.vi"("Name"=w400) -> ("String"=w398:string)  [unwired: 9 in, 1 out]
            n203 = Equal?(x="Both directions", y=w398) -> (x = y?=w396:bool)
            n204 = Not(x=w396) -> (.not. x?=w397:bool)
            n205 = property on="Rev/Fwd" class="Clust (strict)"("Visible"=w396) -> ()  [unwired: 2 in, 2 out]
            n206 = property on="On/Off" class="Bool (strict)"("Visible"=w397, "Caption.Text"=w395) -> ()  [unwired: 2 in, 2 out]
          }
          frame "Compressor", "Digital Out" {
            w403 = FALSE ("Visible")
            # "Get direction and finish"
            n207 = property on="Motor" class="Clust (strict)"("Visible"=w403) -> ()  [unwired: 2 in, 2 out]
            n208 = property on="Test Slider" class="Slide (strict)"("Visible"=w403) -> ()  [unwired: 2 in, 2 out]
            n209 = property on="Test Ring" class="Ring (strict)"("Visible"=w403) -> ()  [unwired: 2 in, 2 out]
            n210 = property on="On/Off" class="Bool (strict)"("Visible"=TRUE, "Caption.Text"=w404) -> ()  [unwired: 2 in, 2 out]
            n211 = property on="Rev/Fwd" class="Clust (strict)"("Visible"=FALSE) -> ()  [unwired: 2 in, 2 out]
          }
          frame "Camera" {
            n212 = call <vilib>:"Get Last Path Segment.vi"("String in"=w411) -> ("String out"=w412:string)  [unwired: 10 in]
            n213 = property on="On/Off" class="Bool (strict)"("Visible"=FALSE) -> ()  [unwired: 2 in, 2 out]
            n214 = property on="Motor" class="Clust (strict)"("Visible"=FALSE) -> ()  [unwired: 2 in, 2 out]
            n215 = property on="Rev/Fwd" class="Clust (strict)"("Visible"=FALSE) -> ()  [unwired: 2 in, 2 out]
            n216 = case shown="\"White Balance  **\"" w412 {
              tunnel: w411 -> [w418 w427 w436 w445 w454 _ w460]
              tunnel: w410 -> [w416 w424 w433 w442 w451 _ _]
              frame "Size  **" {
                n217 = Index Array(array=w416) -> (element=w415:cluster{string[]})  [unwired: 1 in]
                n218 = call <vilib>:"NT Read String.vi"("Name"=w418) -> ("String"=w417:string)  [unwired: 9 in, 1 out]
                n219 = Unbundle(w415) -> (w413:string[])
                n220 = Match First String(2:w413, 3:w417) -> (0:w414:i32)  [unwired: 1 out]
                n221 = property on="Test Ring" class="Ring (strict)"("Value"=w414, "Strings []"=w413) -> ()  [unwired: 2 in, 2 out]
                n222 = property on="Test Ring" class="Ring (strict)"("Visible"=TRUE) -> ()  [unwired: 2 in, 2 out]
                n223 = property on="Test Slider" class="Slide (strict)"("Visible"=FALSE) -> ()  [unwired: 2 in, 2 out]
              }
              frame "White Balance  **" {
                n224 = Index Array(array=w424, index=1) -> (element=w425:cluster{string[]})
                n225 = call <vilib>:"NT Read String.vi"("Name"=w427) -> ("String"=w426:string)  [unwired: 9 in, 1 out]
                n226 = Unbundle(w425) -> (w422:string[])
                n227 = Match First String(2:w422, 3:w426) -> (0:w421:i32)  [unwired: 1 out]
                n228 = property on="Test Ring" class="Ring (strict)"("Value"=w421, "Strings []"=w422) -> ()  [unwired: 2 in, 2 out]
                n229 = property on="Test Ring" class="Ring (strict)"("Visible"=TRUE) -> ()  [unwired: 2 in, 2 out]
                n230 = property on="Test Slider" class="Slide (strict)"("Visible"=FALSE) -> ()  [unwired: 2 in, 2 out]
              }
              frame "Exposure  **" {
                n231 = Index Array(array=w433, index=2) -> (element=w434:cluster{string[]})
                n232 = call <vilib>:"NT Read String.vi"("Name"=w436) -> ("String"=w435:string)  [unwired: 9 in, 1 out]
                n233 = Unbundle(w434) -> (w430:string[])
                n234 = Match First String(2:w430, 3:w435) -> (0:w431:i32)  [unwired: 1 out]
                n235 = property on="Test Ring" class="Ring (strict)"("Value"=w431, "Strings []"=w430) -> ()  [unwired: 2 in, 2 out]
                n236 = property on="Test Ring" class="Ring (strict)"("Visible"=TRUE) -> ()  [unwired: 2 in, 2 out]
                n237 = property on="Test Slider" class="Slide (strict)"("Visible"=FALSE) -> ()  [unwired: 2 in, 2 out]
              }
              frame "Exposure Priority  **" {
                n238 = Index Array(array=w442, index=3) -> (element=w443:cluster{string[]})
                n239 = call <vilib>:"NT Read String.vi"("Name"=w445) -> ("String"=w444:string)  [unwired: 9 in, 1 out]
                n240 = Unbundle(w443) -> (w439:string[])
                n241 = Match First String(2:w439, 3:w444) -> (0:w440:i32)  [unwired: 1 out]
                n242 = property on="Test Ring" class="Ring (strict)"("Value"=w440, "Strings []"=w439) -> ()  [unwired: 2 in, 2 out]
                n243 = property on="Test Ring" class="Ring (strict)"("Visible"=TRUE) -> ()  [unwired: 2 in, 2 out]
                n244 = property on="Test Slider" class="Slide (strict)"("Visible"=FALSE) -> ()  [unwired: 2 in, 2 out]
              }
              frame "Color Enable  **" {
                n245 = Index Array(array=w451, index=4) -> (element=w452:cluster{string[]})
                n246 = call <vilib>:"NT Read String.vi"("Name"=w454) -> ("String"=w453:string)  [unwired: 9 in, 1 out]
                n247 = Unbundle(w452) -> (w448:string[])
                n248 = Match First String(2:w448, 3:w453) -> (0:w449:i32)  [unwired: 1 out]
                n249 = property on="Test Ring" class="Ring (strict)"("Value"=w449, "Strings []"=w448) -> ()  [unwired: 2 in, 2 out]
                n250 = property on="Test Ring" class="Ring (strict)"("Visible"=TRUE) -> ()  [unwired: 2 in, 2 out]
                n251 = property on="Test Slider" class="Slide (strict)"("Visible"=FALSE) -> ()  [unwired: 2 in, 2 out]
              }
              frame Default {
                n252 = property on="Test Ring" class="Ring (strict)"("Visible"=FALSE) -> ()  [unwired: 2 in, 2 out]
                n253 = property on="Test Slider" class="Slide (strict)"("Visible"=FALSE) -> ()  [unwired: 2 in, 2 out]
              }
              frame "Brightness  **", "Color Level  **", "Compression  **", "FPS  **", "Sharpness  **" {
                n254 = call <vilib>:"NT Read Number.vi"("Name"=w460) -> ("Numeric"=w459:dbl)  [unwired: 9 in, 1 out]
                n255 = local write "Test Slider"(w459) -> ()
                n256 = property on="Test Slider" class="Slide (strict)"("Visible"=TRUE, "Scale.Maximum"=100.0 ("Scale.Range:Maximum")) -> ()  [unwired: 2 in, 2 out]
                n257 = property on="Test Ring" class="Ring (strict)"("Visible"=FALSE) -> ()  [unwired: 2 in, 2 out]
              }
            }
          }
        }
        n258 = property on="Progress" class="Clust (strict)"("Visible"=FALSE) -> ()  [unwired: 2 in, 2 out]
      }
      event "Test Name": Mouse Enter {
        # "Populate the ring with the list of tests"
        n259 = event-data() -> ()  [unwired: 1 in, 1 out]
        n260 = call <vilib>:"NT Read String Array.vi"("Name"="TestMode/TestList") -> ("String Array"=w468:string[])  [unwired: 9 in, 1 out]
        n261 = Build Array (concatenate)("Select the test to run...", w468) -> (w467:string[])
        n262 = property on="Test Name" class="Ring (strict)"("Strings []"=w467) -> ()  [unwired: 2 in, 2 out]
      }
      event "Test Name": Value Change {
        w470 = FALSE ("Visible")
        # "Tell the robot the test name to run"
        n263 = event-data() -> ("NewVal"=w474:u16)  [unwired: 1 in]
        n264 = property on="Test Name" class="Ring (strict)"() -> ("Strings []"=w475:string[])  [unwired: 2 in, 2 out]
        n265 = local write "Progress"(T6 {"Test Progress"=0, "Test Progress Text"=""} ("Progress")) -> ()
        n266 = Index Array(array=w475, index=w474) -> (element=w473:string)
        n267 = call <vilib>:"NT Write String.vi"("String"=w473, "Name"="TestMode/TestName") -> ()  [unwired: 9 in, 1 out]
        n268 = property on="Progress" class="Clust (strict)"("Visible"=TRUE) -> ()  [unwired: 2 in, 2 out]
        n269 = property on="Motor" class="Clust (strict)"("Visible"=w470) -> ()  [unwired: 2 in, 2 out]
        n270 = property on="Test Slider" class="Slide (strict)"("Visible"=w470) -> ()  [unwired: 2 in, 2 out]
        n271 = property on="On/Off" class="Bool (strict)"("Visible"=w470) -> ()  [unwired: 2 in, 2 out]
        n272 = property on="Rev/Fwd" class="Clust (strict)"("Visible"=w470) -> ()  [unwired: 2 in, 2 out]
        n273 = property on="Test Ring" class="Ring (strict)"("Visible"=w470) -> ()  [unwired: 2 in, 2 out]
      }
      event "Select Auto": Mouse Enter {
        # "Populate the combo box with the list of autonomous options"
        n274 = event-data() -> ()  [unwired: 1 in, 1 out]
        n275 = call <vilib>:"NT Read String Array.vi"("Name"="Auto List") -> ("String Array"=w477:string[])  [unwired: 9 in, 1 out]
        n276 = property on="Select Auto" class="CmbBox"("Strings[]"=w477) -> ()  [unwired: 2 in, 2 out]
      }
      event "Select Auto": Value Change {
        # "User modified the Auto Selection. Write to NT variable so robot knows."
        n277 = event-data() -> ("NewVal"=w480:string)  [unwired: 1 in]
        n278 = call <vilib>:"NT Write String.vi"("String"=w480, "Name"="Auto Selector") -> ()  [unwired: 9 in, 1 out]
      }
      event "Command Selection": Value Change {
        # "Get the params and show in table"
        n279 = event-data() -> ("NewVal"=w486:i32)  [unwired: 1 in]
        n280 = property on="Command Selection" class="MCListbox (strict)"() -> ("ItemNames"=w484:string[][])  [unwired: 2 in, 2 out]
        n281 = call <vilib>:"WPI_DashboardUpdate Command Params.vi"("NewVal"=w486, "Commands"=w484, "Param Tbl"=w485) -> ()  [unwired: 8 in, 1 out]
      }
      event "Execute Command": Value Change {
        # "Started one, Unique ID holds\nresponse"
        n282 = event-data() -> ()  [unwired: 1 in, 1 out]
        n283 = property on="Command Selection" class="MCListbox (strict)"() -> ("ItemNames"=w497:string[][])  [unwired: 2 in, 2 out]
        n284 = Index Array(array=w497, index (row)="Command Selection", index (col)=0) -> (element=w495:string)
        n285 = call <vilib>:"Invoke Commands.vi"("Command Params"="Command Params", "Function Name"=w495) -> ("Params"=w491:u8, "Started"=w490:bool)  [unwired: 7 in, 1 out]
        n286 = Array Subset(array="Command Params", length (row)=w491) -> (w492:string[][])  [unwired: 3 in]
        n287 = Select(t="Executing" ("Cmd Status"), s=w490, f="" ("Cmd Status")) -> (s? t:f=→"Cmd Status":string)
      }
      event "Command Selection": Double Click {
        n288 = event-data() -> ("Row"=w505:i32)  [unwired: 1 in]
        n289 = property on="Command Selection" class="MCListbox (strict)"() -> ("ItemNames"=w508:string[][])  [unwired: 2 in, 2 out]
        n290 = local read "Command Params"() -> (w504:string[][])
        n291 = Index Array(array=w508, index (row)=w505, index (col)=0) -> (element=w506:string)
        n292 = call <vilib>:"Invoke Commands.vi"("Command Params"=w504, "Function Name"=w506) -> ("Params"=w503:u8, "Started"=w498:bool)  [unwired: 7 in, 1 out]
        n293 = Array Subset(array=w504, length (row)=w503) -> (w502:string[][])  [unwired: 3 in]
        n294 = Select(t="Executing" ("Cmd Status"), s=w498, f="" ("Cmd Status")) -> (s? t:f=w499:string)
        n295 = local write "Cmd Status"(w499) -> ()
      }
      event "CheckList": Double Click {
        # "Shift clears all"
        # "Update symbols on the listbox"
        n296 = event-data() -> ("PlatMods.Shift"=w510:bool, "Row"=w512:i32)  [unwired: 1 in]
        n297 = case shown="True" w510 {
          tunnel: w512 -> [w516 _]
          tunnel: 1 -> [w515 _]
          frame False {
            n298 = property on="CheckList" class="LstBox (strict)"() -> ("Item Symbols"=w514:i32[])  [unwired: 2 in, 2 out]
            n299 = Replace Array Subset(array=w514, new element=w515, index=w516) -> (w513:i32[])
            n300 = property on="CheckList" class="LstBox (strict)"("Item Symbols"=w513) -> ()  [unwired: 2 in, 2 out]
          }
          frame True {
            w517 = 0 ("Top Row")
            n301 = property on="CheckList" class="LstBox (strict)"() -> ("Number of Rows"=w519:u32)  [unwired: 2 in, 2 out]
            n302 = Initialize Array(0, w519) -> (w518:i32[])
            n303 = property on="CheckList" class="LstBox (strict)"("Top Row"=w517, "Value"=w517, "Item Symbols"=w518) -> ()  [unwired: 2 in, 2 out]
          }
        }
      }
      event "CheckList": Key Down {
        # "Update symbols on the listbox\nLeft and right keys check and uncheck"
        n304 = event-data() -> ("VKey"=w523:T23)  [unwired: 1 in]
        n305 = case shown="\"Left\", \"Right\"" w523 {
          selector: w523 -> [w528 _]
          tunnel: eventvkey."Left" ("VKey") -> [w526 _]
          frame "Left", "Right" {
            n306 = Equal?(x=w526, y=w528) -> (x = y?=w527:bool)
            n307 = Select(t=0, s=w527, f=1) -> (s? t:f=w529:i32)
            n308 = property on="CheckList" class="LstBox (strict)"() -> ("Item Symbols"=w532:i32[])  [unwired: 2 in, 2 out]
            n309 = Replace Array Subset(array=w532, new element=w529, index="CheckList") -> (w531:i32[])
            n310 = property on="CheckList" class="LstBox (strict)"("Item Symbols"=w531) -> ()  [unwired: 2 in, 2 out]
          }
          frame Default {
          }
        }
      }
      event "Motor.Enable": Value Change {
        # "When the test mode otor enable helper is set, update that\ntree row item's value"
        n311 = event-data() -> ("NewVal"=w538:bool)  [unwired: 1 in]
        n312 = Unbundle("Motor") -> ("Value"=w537:dbl)  [unwired: 1 out]
        n313 = Select(t=w537, s=w538, f=0.0) -> (s? t:f=w535:dbl)
        n314 = call <vilib>:"NT Write Number.vi"("Numeric"=w535, "Name"=w534) -> ()  [unwired: 9 in, 1 out]
      }
      event "Test Slider": Value Change {
        # "When the test mode slider helper is set, update that\ntree row item's value"
        n315 = event-data() -> ("NewVal"=w541:dbl)  [unwired: 1 in]
        n316 = call <vilib>:"NT Write Number.vi"("Numeric"=w541, "Name"=w542) -> ()  [unwired: 9 in, 1 out]
      }
      event "On/Off": Value Change {
        # "When the test mode on/off helper value is set, update that\ntree row item's value"
        n317 = event-data() -> ("NewVal"=w546:bool)  [unwired: 1 in]
        n318 = Boolean To (0,1)(Boolean=w546) -> (0, 1=w545:i16)
        n319 = call <vilib>:"NT Write Number.vi"("Numeric"=w545, "Name"=w544) -> ()  [unwired: 9 in, 1 out]
      }
      event "Rev/Fwd": Value Change {
        # "When the test mode helper value for relays is set, update that\ntree row item's value"
        n320 = event-data() -> ("NewVal.Forward"=w554:bool, "NewVal.Reverse"=w553:bool)  [unwired: 1 in]
        n321 = Boolean To (0,1)(Boolean=w554) -> (0, 1=w550:i16)
        n322 = Boolean To (0,1)(Boolean=w553) -> (0, 1=w552:i16)
        n323 = Negate(x=w552) -> (-x=w551:i16)
        n324 = Add(x=w550, y=w551) -> (x+y=w549:i16)
        n325 = call <vilib>:"NT Write Number.vi"("Numeric"=w549, "Name"=w548) -> ()  [unwired: 9 in, 1 out]
      }
      event "Test Ring": Value Change {
        # "When a test mode helper value is selected from the ring,\nset the tree item's variable to the string value"
        n326 = event-data() -> ("NewVal"=w558:u16)  [unwired: 1 in]
        n327 = property on="Test Ring" class="Ring (strict)"() -> ("Strings []"=w559:string[])  [unwired: 2 in, 2 out]
        n328 = Index Array(array=w559, index=w558) -> (element=w557:string)
        n329 = call <vilib>:"NT Write String.vi"("String"=w557, "Name"=w556) -> ()  [unwired: 9 in, 1 out]
      }
      event "Rec Mode": Value Change {
        # "Update globals for recording mode and path to read log from.\nClear when logging and let NetworkTables set path for vision to\nuse."
        n330 = event-data() -> ("NewVal"=w570:enum32{"Stop", "Record", "Playback"})  [unwired: 1 in]
        n331 = global write "WPI_DashboardLogging Global.vi" "Logging Filename"(path "") -> ()
        n332 = global write "WPI_DashboardLogging Global.vi" "Recording"(w570) -> ()
        n333 = case shown="\"Playback\"" w570 {
          tunnel: w569 -> [_ w572 w581]
          tunnel: [_ _ w580] -> w567
          tunnel: [_ _ w579] -> _
          tunnel: w565 -> [_ _ w577]
          tunnel: cluster{i32, i32} {-250, 170} -> [_ _ w576]
          tunnel: [_ _ T24 {"Image Size"=TRUE, "Image Type"=TRUE, "Pixel Value"=TRUE, "ROI Information"=TRUE, "Zoom Factor"=FALSE} ("Image Information Shown:All Elements")] -> w560
          tunnel: [_ _ TRUE ("Zoom Factor")] -> w561
          tunnel: w563 -> [_ _ w573]
          frame Default {
          }
          frame "Stop", "Record" {
            # "Place Window too"
            n334 = invoke class="VI" method="FP.Close"(reference=w572) -> (reference out=w571:refnum<vi>)  [unwired: 2 in, 2 out]
            n335 = invoke class="VI" method="Abort VI"(reference=w571) -> ()  [unwired: 2 in, 3 out]
          }
          frame "Playback" {
            n336 = call "Open Playback Panel.vi"("Offset"=w576, "DB VI Ref"=w577, "Playback in"=w581) -> ("Playback out"=w578:refnum<vi>)  [unwired: 8 in]
            n337 = register-events(w578, w573) -> (reference out=w580:refnum<event-registration>, error out=w579:errorcluster)  [unwired: 2 in]
          }
        }
        n338 = property on="Camera Image Right" class="ImageControl"("Image Information Shown"=w560, "Image Information Visible"=w561) -> ()  [unwired: 2 in, 2 out]
        n339 = property on="Camera Image" class="ImageControl"("Image Information Shown"=w560, "Image Information Visible"=w561) -> ()  [unwired: 2 in, 2 out]
        n340 = call <vilib>:"WPI_DashboardNT Log FieldName Cache.vi"("Operation"=enum16{"Lookup/Add", "Index", "Clear"}."Clear") -> ()  [unwired: 8 in, 3 out]
      }
      event Panel Close {
        w583 = enum32{"Stop", "Record", "Playback"}."Stop" ("Rec Mode")
        # "Playback window has been closed, abort"
        n341 = event-data() -> ()  [unwired: 1 in, 4 out]
        n342 = local write "Rec Mode"(w583) -> ()
        n343 = global write "WPI_DashboardLogging Global.vi" "Recording"(w583) -> ()
      }
      event Panel Close {
        # "Abort playback window and ourself"
        n344 = event-data() -> ()  [unwired: 1 in, 4 out]
        n345 = invoke class="VI" method="FP.Close"(reference=w587) -> (reference out=w586:refnum<vi>)  [unwired: 2 in, 2 out]
        n346 = invoke class="VI" method="Abort VI"(reference=w586) -> (error out=w585:errorcluster)  [unwired: 2 in, 2 out]
        n347 = invoke class="VI" method="Abort VI"(error in=w585) -> ()  [unwired: 2 in, 3 out]
      }
      event User Event {
        n348 = event-data() -> ("IDs"=w594:cluster{"RPC field ID":u16, "Unique ID":u16}, "String"=w593:string)  [unwired: 1 in]
        n349 = Bundle("IDs"=w594, "String"=w593) -> (w592:T9)  [unwired: 1 in]
        n350 = call <vilib>:"Retrieve RPC Response.vi"("RPC Response"=w592) -> ("Output"=w590:string[][])  [unwired: 10 in]
        n351 = Build Array (concatenate)(w588, w590) -> (w589:string[][])
        n352 = local write "Command Params"(w589) -> ()
        n353 = local write "Cmd Status"("" ("Cmd Status")) -> ()
      }
      event "Tree": Double Click {
        n354 = event-data() -> ("PlatMods"=w600:T27, "Tag"=w597:string)  [unwired: 1 in]
        n355 = Unbundle(w600) -> ("Shift"=w599:bool)  [unwired: 4 out]
        n356 = String Subset(string=w597, length (rest)=1 ("length (rest)")) -> (substring=w596:string)  [unwired: 1 in]
        n357 = Not(x=w599) -> (.not. x?=w598:bool)
        n358 = case shown="\"/\"" w596 {
          tunnel: w597 -> [_ w603]
          tunnel: w598 -> [_ w602]
          frame Default {
          }
          frame "/" {
            n359 = call <vilib>:"NT Update Persistence.vi"("Persistence"=w602, "Name"=w603) -> ()  [unwired: 9 in, 1 out]
          }
        }
      }
    }
  }
  n360 = while {
    tunnel: w65 -> [w605]
    i -> [w608]
    stop <- FALSE stop-if-true
    n361 = Wait (ms)(milliseconds to wait=u32 100) -> ()  [unwired: 1 out]
    n362 = case shown="\"Playback\"" "Rec Mode" {
      tunnel: w608 -> [_ _ w623]
      tunnel: [u32 2829099 ("Base Color") u32 11141120 ("Target Color") w612] -> w604
      frame "Stop", Default {
        # "Reset the color, extra updates don't cost much"
      }
      frame "Record" {
      }
      frame "Playback" {
        # "Playback"
        n363 = Quotient & Remainder(x=w623, y=u32 50 ("milliseconds to wait")) -> (x-y*floor(x/y)=w619:u32)  [unwired: 1 out]
        n364 = Divide(x=w619, y=u32 50 ("milliseconds to wait")) -> (x/y=w616:dbl)
        n365 = Multiply(x=6.283185307179586, y=w616) -> (x*y=w621:dbl)
        n366 = Sine(x=w621) -> (sin(x)=w620:dbl)
        n367 = Absolute Value(x=w620) -> (abs(x)=w613:dbl)
        n368 = call "Interpolate RGB Color.vi"("Proportion"=w613, "Target Color"=u32 30976, "Base Color"=u32 2829099) -> ("Result Color"=w612:u32)  [unwired: 8 in]
      }
    }
    n369 = property class="Pane"(reference=w605, "PaneColor"=w604) -> ()  [unwired: 1 in, 2 out]
  }
  n370 = local write "Dashboard Tab"(T2."Drive" ("Dashboard Tab")) -> ()
  n371 = property on="On/Off" class="Bool (strict)"("Visible"=w36) -> ()  [unwired: 2 in, 2 out]
  n372 = property on="Motor" class="Clust (strict)"("Visible"=w36) -> ()  [unwired: 2 in, 2 out]
  n373 = property on="Progress" class="Clust (strict)"("Visible"=w36) -> ()  [unwired: 2 in, 2 out]
  n374 = property on="Test Ring" class="Ring (strict)"("Visible"=w36) -> ()  [unwired: 2 in, 2 out]
  n375 = property on="Rev/Fwd" class="Clust (strict)"("Visible"=w36) -> ()  [unwired: 2 in, 2 out]
  n376 = local write "Command Selection"(u16 0 ("milliseconds to wait")) -> ()
  n377 = while {
    tunnel: u16 1741 ("timeout ms (25000)") -> [w625]
    stop <- FALSE stop-if-true
    n378 = TCP Create Listener(10:w625) -> (0:w624:errorcluster, 3:w626:refnum<k5>)  [unwired: 4 in, 1 out]
    n379 = case shown="No Error" w624 {
      selector: w624 -> [w628 _]
      tunnel: w626 -> [w629 _]
      frame No Error {
        n380 = while {
          tunnel: w629 -> [w632]
          tunnel: w628 -> [w631]
          stop <- FALSE stop-if-true
          n381 = TCP Wait On Listener(8:w631, 11:w632) -> (0:w633:errorcluster, 4:w634:refnum<k5>)  [unwired: 2 in, 3 out]
          n382 = local write "TCP"(w634) -> ()
          n383 = case shown="No Error" w633 {
            frame No Error {
            }
            frame Error {
              n384 = Wait (ms)(milliseconds to wait=u32 1000) -> ()  [unwired: 1 out]
            }
          }
        }
      }
      frame Error {
        n385 = Wait (ms)(milliseconds to wait=u32 1000) -> ()  [unwired: 1 out]
      }
    }
  }
  n386 = local write "Command Params"(string[][] [] ("Command Params")) -> ()
  n387 = global write "WPI_DashboardLogging Global.vi" "Recording"(w59) -> ()
  n388 = local write "Rec Mode"(w59) -> ()
  n389 = call <vilib>:"NT Write String.vi"("String"="Select Auto", "Name"="Auto Selector") -> ()  [unwired: 9 in, 1 out]
